vi "Resistivity of Bar sample Test.vi"(8 "error in (no error)":errorcluster) -> (0 "error out":errorcluster)   [LabVIEW 2016, in "Hall Effect Library.lvlib"]
doc: "This VI executes the Van Der Pauw Resisitivty Test and returns the voltage measurements V1-V8 taken during the test."
uses:
  Hall Effect Library.lvlib
  Controls/Measurement.ctl
  Public/Controls/Data Items.ctl
  Public/Controls/Tests.ctl
  Global Variables/Test Settings.vi
  Global Variables/Instrument Locations.vi
  Global Variables/Hall Effect Data.vi
panel:
  out "Soak Until":timestamp
  out "Measurement":T1
  out "Test Step":T2(ring)
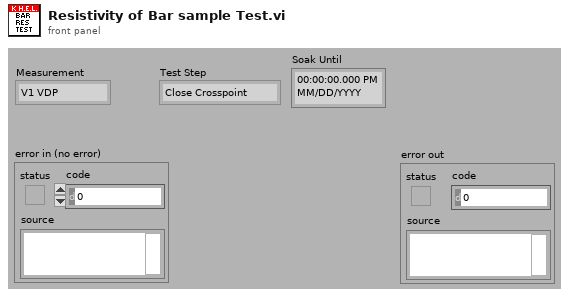
[diagram p1: front panel]
types:
  T1 = typedef "Hall Effect Library.lvlib/Measurement.ctl" = enum16{"V1 VDP", "V2 VDP", "V3 VDP", "V4 VDP", "V5 VDP", "V6 VDP", "V7 VDP", "V8 VDP", "V1 HE", "V2 HE", "V3 HE", "V4 HE", "V5 HE", "V6 HE", "V7 HE", "V8 HE", "V1 Res Bar", "V1 Hall Bar", "V1 Res 6-Cot", "V2 Res 6-Cot", "V3 Res 6-Cot", "V4 Res 6-Cot", "V1 Hall 6-Cot", "V2 Hall 6-Cot", "V3 Hall 6-Cot", "V4 Hall 6-Cot", "V5 Hall 6-Cot", "V6 Hall 6-Cot", "V7 Hall 6-Cot", "V8 Hall 6-Cot", "V1 Res 8-Cot", "V2 Res 8-Cot", "V3 Res 8-Cot", "V4 Res 8-Cot", "V1 Hall 8-Cot", "V2 Hall 8-Cot", "V3 Hall 8-Cot", "V4 Hall 8-Cot"}
  T2 = enum16{"Close Crosspoint", "Soak 1", "Zero Ammeter", "Zero Voltmeter", "I-SRC On", "Init Ammeter", "Soak 2", "Measure I", "Measure V", "I-SRC Off", "Open Crosspoint", "Done"}
  T3 = typedef "Hall Effect Library.lvlib/Resisitivity.ctl" = enum16{"Low", "High"}
  T4 = typedef "Hall Effect Library.lvlib/Tests.ctl" = enum16{"Van Der Pauw", "Hall Effect", "Bar Sample Resistivity", "Bar Sample Hall ", "6-Contact Sample Resistivity", "6-Contact Sample Hall", "8-Contact Sample Resistivity", "8-Contact Sample Hall", ""}
  T5 = typedef "Hall Effect Library.lvlib/Data Items.ctl" = enum16{"V1 Van Der Pauw", "V2 Van Der Pauw", "V3 Van Der Pauw", "V4 Van Der Pauw", "V5 Van Der Pauw", "V6 Van Der Pauw", "V7 Van Der Pauw", "V8 Van Der Pauw", "V1 Hall Effect", "V2 Hall Effect", "V3 Hall Effect", "V4 Hall Effect", "V5 Hall Effect", "V6  Hall Effect", "V7 Hall Effect", "V8 Hall Effect", "V1 Res Bar", "V1 Hall Bar", "V1 Res 6-Cot", "V2 Res 6-Cot", "V3 Res 6-Cot", "V4 Res 6-Cot", "V1 Hall 6-Cot", "V2 Hall 6-Cot", "V3 Hall 6-Cot", "V4 Hall 6-Cot", "V5 Hall 6-Cot", "V6 Hall 6-Cot", "V7 Hall 6-Cot", "V8 Hall 6-Cot", "V1 Res 8-Cot", "V2 Res 8-Cot", "V3 Res 8-Cot", "V4 Res 8-Cot", "V1 Hall 8-Cot", "V2 Hall 8-Cot", "V3 Hall 8-Cot", "V4 Hall 8-Cot", "Van Der Pauw Results", "Hall Effect Results", "Bar Sample Resistivity Results", "Bar Sample Hall Results", "6-Contact Resistivity Results", "6-Contact Hall Results", "8-Contact Resistivity Results", "8-Contact Hall Results"}
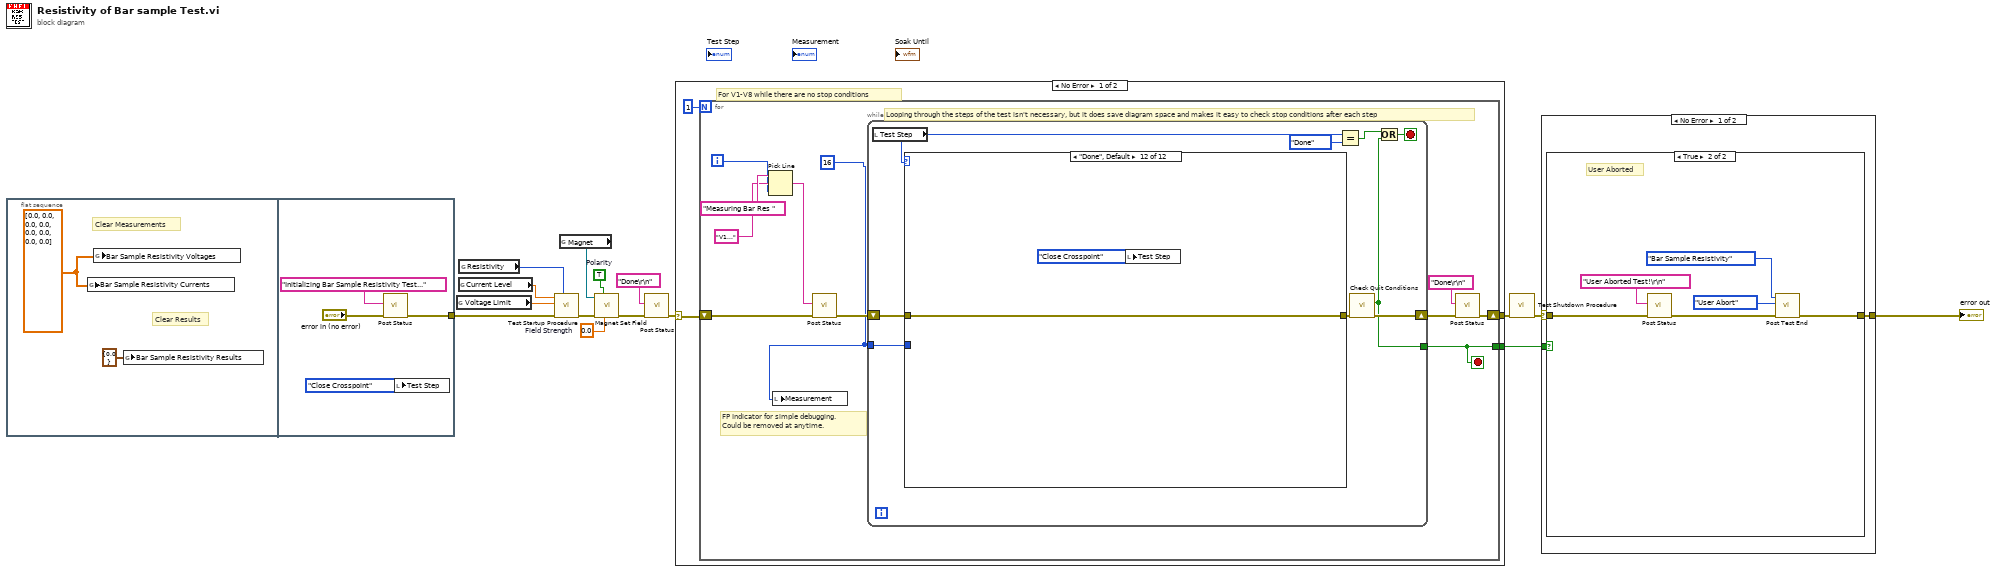
[diagram p0: block diagram]
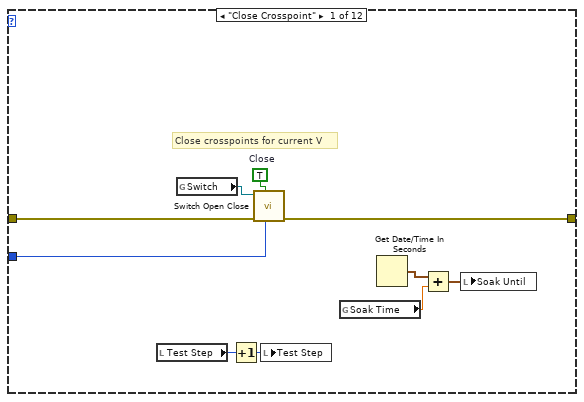
[diagram p2: hidden frame]
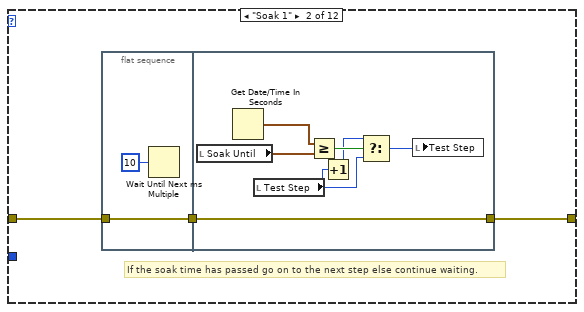
[diagram p3: hidden frame]
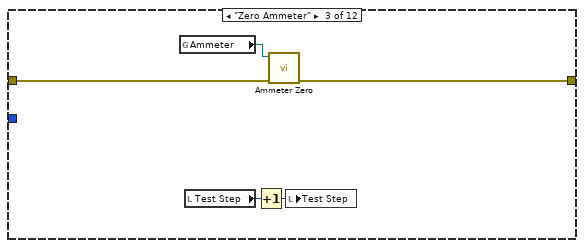
[diagram p4: hidden frame]
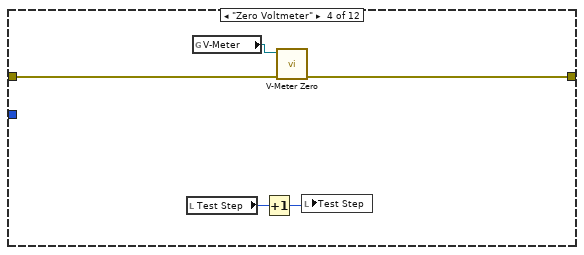
[diagram p5: hidden frame]
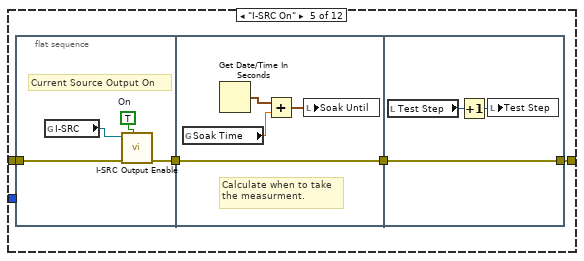
[diagram p6: hidden frame]
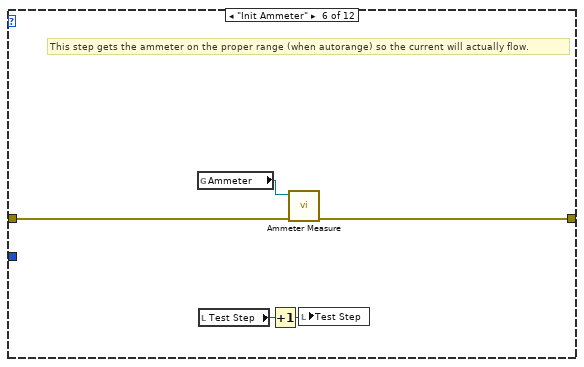
[diagram p7: hidden frame]
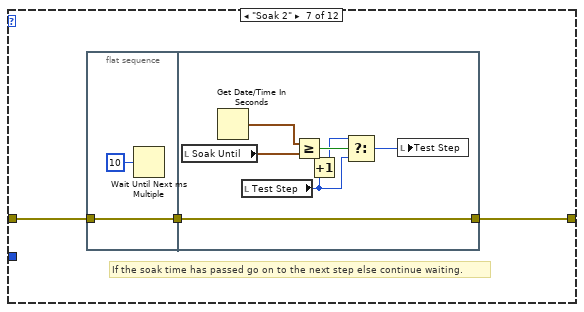
[diagram p8: hidden frame]
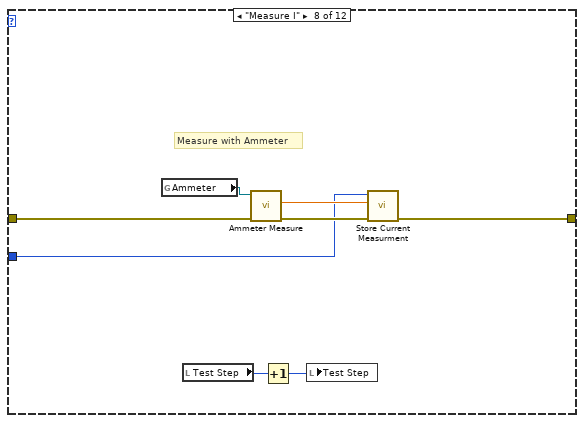
[diagram p9: hidden frame]
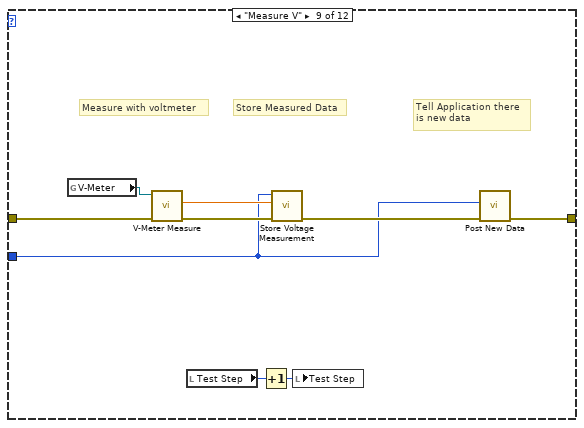
[diagram p10: hidden frame]
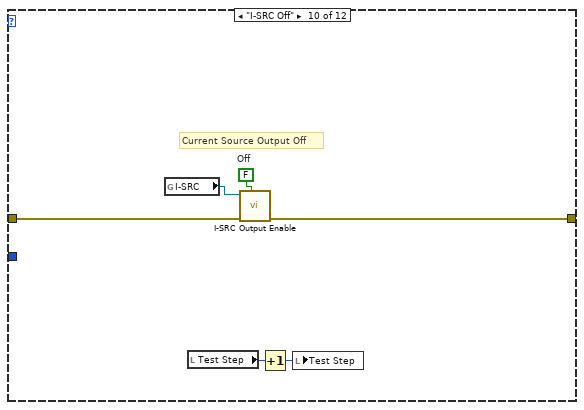
[diagram p11: hidden frame]
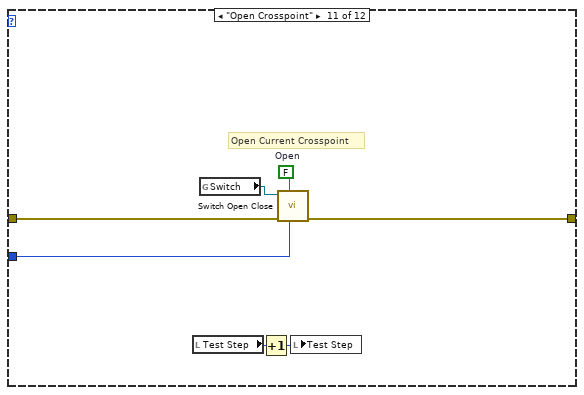
[diagram p12: hidden frame]
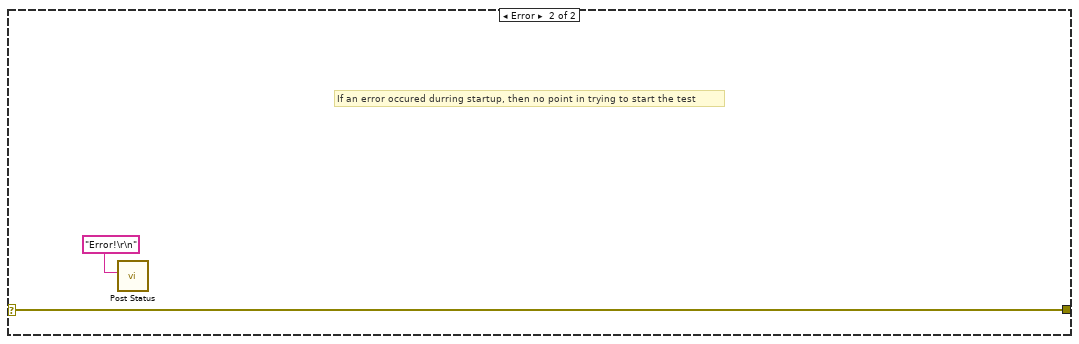
[diagram p13: hidden frame]
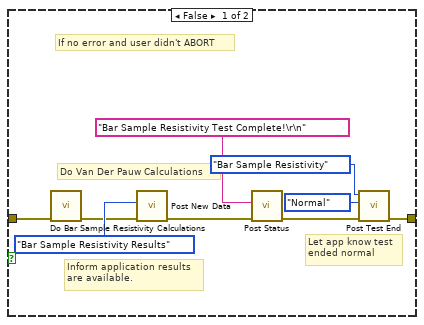
[diagram p14: hidden frame]
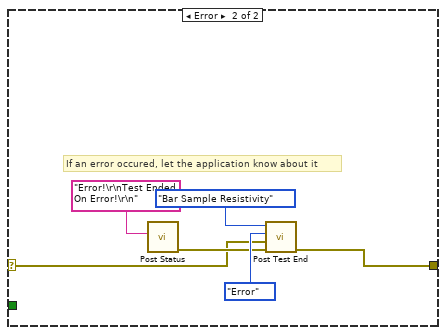
[diagram p15: hidden frame]
diagram:
  w4 = TRUE  # Polarity
  w5 = 0.0  # Field Strength
  n1 = flat-sequence {
    tunnel: [w21] -> w7
    frame #0 {
      w17 = dbl[] [0.0, 0.0, 0.0, 0.0, 0.0, 0.0, 0.0, 0.0] ("Van Der Pauw Voltages")
      # "Clear Results"
      # "Clear Measurements"
      n2 = global write "Hall Effect Data.vi" "Bar Sample Resistivity Currents"(w17) -> ()
      n3 = global write "Hall Effect Data.vi" "Bar Sample Resistivity Voltages"(w17) -> ()
      n4 = global write "Hall Effect Data.vi" "Bar Sample Resistivity Results"(cluster{"p":dbl} {"p"=0.0} ("Bar Sample Resistivity Results")) -> ()
    }
    frame #1 {
      n5 = call "Post Status.vi"("error in (no error)"="error in (no error)", "Status Message"="Initializing Bar Sample Resistivity Test...") -> ("error out"=w21:errorcluster)  [unwired: 9 out]
      n6 = local write "Test Step"(T2."Close Crosspoint" ("Test Step")) -> ()
    }
  }
  n7 = global read "Test Settings.vi" "Voltage Limit"() -> (w8:dbl)
  n8 = global read "Test Settings.vi" "Current Level"() -> (w9:dbl)
  n9 = global read "Test Settings.vi" "Resistivity"() -> (w10:T3)
  n10 = call "Test Startup Procedure.vi"("Resistivity"=w10, "error in (no error)"=w7, "Voltage Limit"=w8, "Current Level"=w9) -> ("error out"=w2:errorcluster)  [unwired: 7 out]
  n11 = global read "Instrument Locations.vi" "Magnet"() -> (w3:refnum<visa-resource-name>)
  n12 = call "Magnet Set Field.vi"("Field Strength"=w5, "Polarity"=w4, "error in (no error)"=w2, "VISA resource name in"=w3) -> ("error out"=w1:errorcluster)  [unwired: 7 out]
  n13 = call "Post Status.vi"("error in (no error)"=w1, "Status Message"="Done\r\n") -> ("error out"=w12:errorcluster)  [unwired: 9 out]
  n14 = case shown="No Error" w12 {
    selector: w12 -> [w23 w143]
    tunnel: [w25 w143] -> w11
    tunnel: [w24 _] -> w13
    frame No Error {
      # "For V1-V8 while there are no stop conditions"
      n15 = for {
        N: 1 -> [_]
        shift-right: [w29] -> w25
        shift-left: w23 -> [w32]
        tunnel: [w28] -> w24
        i -> [w27]
        stop <- w28 stop-if-true
        w26 = 16
        # "FP Indicator for simple debugging.\nCould be removed at anytime."
        # "Looping through the steps of the test isn't necessary, but it does save diagram space and makes it easy to check stop conditions after each step"
        n16 = Pick Line(string ("")="Measuring Bar Res ", multi-line string="V1...", line index=w27) -> (output string=w34:string)
        n17 = local write "Measurement"(w26) -> ()
        n18 = call "Post Status.vi"("error in (no error)"=w32, "Status Message"=w34) -> ("error out"=w33:errorcluster)  [unwired: 9 out]
        n19 = while {
          shift-right: [w43] -> w30
          shift-left: w33 -> [w45]
          tunnel: w26 -> [w44]
          tunnel: [w39] -> w28
          stop <- w42 stop-if-true
          n20 = local read "Test Step"() -> (w40:T2)
          n21 = case shown="\"Done\", Default" w40 {
            tunnel: [w53 w56 w70 w75 w80 w96 w99 w114 w121 w129 w137 w141] -> w38
            tunnel: w45 -> [w52 w57 w71 w76 w81 w97 w100 w116 w125 w130 w136 w141]
            tunnel: w44 -> [w51 _ _ _ _ _ _ w112 w120 _ w135 _]
            frame "Close Crosspoint" {
              w54 = TRUE  # Close
              # "Close crosspoints for current V"
              n22 = local read "Test Step"() -> (w47:T2)
              n23 = global read "Instrument Locations.vi" "Switch"() -> (w55:refnum<visa-resource-name>)
              n24 = Increment(x=w47) -> (x+1=w46:T2)
              n25 = call "Switch Open Close.vi"("Measurement"=w51, "Open/Close (F: Open)"=w54, "error in (no error)"=w52, "VISA resource name in"=w55) -> ("error out"=w53:errorcluster)  [unwired: 7 out]
              n26 = local write "Test Step"(w46) -> ()
              n27 = global read "Test Settings.vi" "Soak Time"() -> (w49:dbl)
              n28 = Get Date/Time In Seconds() -> (seconds since 1Jan1904=w48:timestamp)
              n29 = Add(x=w48, y=w49) -> (x+y=w50:timestamp)
              n30 = local write "Soak Until"(w50) -> ()
            }
            frame "Soak 1" {
              # "If the soak time has passed go on to the next step else continue waiting."
              n31 = flat-sequence {
                tunnel: w57 -> [w59]
                tunnel: [w59] -> w58
                tunnel: [w63] -> w56
                tunnel: w58 -> [w63]
                frame #0 {
                  n32 = Wait Until Next ms Multiple(millisecond multiple=u32 10) -> ()  [unwired: 1 out]
                }
                frame #1 {
                  n33 = local read "Soak Until"() -> (w66:timestamp)
                  n34 = Get Date/Time In Seconds() -> (seconds since 1Jan1904=w67:timestamp)
                  n35 = local read "Test Step"() -> (w62:T2)
                  n36 = Greater Or Equal?(x=w67, y=w66) -> (x >= y?=w65:bool)
                  n37 = Increment(x=w62) -> (x+1=w61:T2)
                  n38 = Select(t=w61, s=w65, f=w62) -> (s? t:f=w64:T2)
                  n39 = local write "Test Step"(w64) -> ()
                }
              }
            }
            frame "Zero Ammeter" {
              n40 = global read "Instrument Locations.vi" "Ammeter"() -> (w72:refnum<visa-resource-name>)
              n41 = local read "Test Step"() -> (w69:T2)
              n42 = Increment(x=w69) -> (x+1=w68:T2)
              n43 = call "Ammeter Zero.vi"("error in (no error)"=w71, "VISA resource name in"=w72) -> ("error out"=w70:errorcluster)  [unwired: 9 out]
              n44 = local write "Test Step"(w68) -> ()
            }
            frame "Zero Voltmeter" {
              n45 = local read "Test Step"() -> (w73:T2)
              n46 = global read "Instrument Locations.vi" "V-Meter"() -> (w77:refnum<visa-resource-name>)
              n47 = Increment(x=w73) -> (x+1=w74:T2)
              n48 = call "V-Meter Zero.vi"("error in (no error)"=w76, "VISA resource name in"=w77) -> ("error out"=w75:errorcluster)  [unwired: 9 out]
              n49 = local write "Test Step"(w74) -> ()
            }
            frame "I-SRC On" {
              n50 = flat-sequence {
                tunnel: w81 -> [w83]
                tunnel: [w82] -> w79
                tunnel: w79 -> [w89]
                tunnel: [w89] -> w78
                tunnel: [w92] -> w80
                tunnel: w78 -> [w92]
                frame #0 {
                  w84 = TRUE  # On
                  # "Current Source Output On"
                  n51 = global read "Instrument Locations.vi" "I-SRC"() -> (w85:refnum<visa-resource-name>)
                  n52 = call "I-SRC Output Enable.vi"("Output (Off)"=w84, "error in (no error)"=w83, "VISA resource name in"=w85) -> ("error out"=w82:errorcluster)  [unwired: 8 out]
                }
                frame #1 {
                  # "Calculate when to take\nthe measurment."
                  n53 = global read "Test Settings.vi" "Soak Time"() -> (w87:dbl)
                  n54 = Get Date/Time In Seconds() -> (seconds since 1Jan1904=w86:timestamp)
                  n55 = Add(x=w86, y=w87) -> (x+y=w88:timestamp)
                  n56 = local write "Soak Until"(w88) -> ()
                }
                frame #2 {
                  n57 = local read "Test Step"() -> (w91:T2)
                  n58 = Increment(x=w91) -> (x+1=w90:T2)
                  n59 = local write "Test Step"(w90) -> ()
                }
              }
            }
            frame "Init Ammeter" {
              # "This step gets the ammeter on the proper range (when autorange) so the current will actually flow."
              n60 = global read "Instrument Locations.vi" "Ammeter"() -> (w95:refnum<visa-resource-name>)
              n61 = local read "Test Step"() -> (w94:T2)
              n62 = Increment(x=w94) -> (x+1=w93:T2)
              n63 = call "Ammeter Measure.vi"("error in (no error)"=w97, "VISA resource name in"=w95) -> ("error out"=w96:errorcluster)  [unwired: 9 out]
              n64 = local write "Test Step"(w93) -> ()
            }
            frame "Soak 2" {
              # "If the soak time has passed go on to the next step else continue waiting."
              n65 = flat-sequence {
                tunnel: w100 -> [w101]
                tunnel: [w101] -> w98
                tunnel: [w105] -> w99
                tunnel: w98 -> [w105]
                frame #0 {
                  n66 = Wait Until Next ms Multiple(millisecond multiple=u32 10) -> ()  [unwired: 1 out]
                }
                frame #1 {
                  n67 = local read "Soak Until"() -> (w108:timestamp)
                  n68 = Get Date/Time In Seconds() -> (seconds since 1Jan1904=w109:timestamp)
                  n69 = local read "Test Step"() -> (w103:T2)
                  n70 = Greater Or Equal?(x=w109, y=w108) -> (x >= y?=w107:bool)
                  n71 = Increment(x=w103) -> (x+1=w104:T2)
                  n72 = Select(t=w104, s=w107, f=w103) -> (s? t:f=w106:T2)
                  n73 = local write "Test Step"(w106) -> ()
                }
              }
            }
            frame "Measure I" {
              # "Measure with Ammeter"
              n74 = global read "Instrument Locations.vi" "Ammeter"() -> (w117:refnum<visa-resource-name>)
              n75 = local read "Test Step"() -> (w111:T2)
              n76 = call "Ammeter Measure.vi"("error in (no error)"=w116, "VISA resource name in"=w117) -> ("error out"=w115:errorcluster, "Measurement"=w113:dbl)  [unwired: 8 out]
              n77 = Increment(x=w111) -> (x+1=w110:T2)
              n78 = local write "Test Step"(w110) -> ()
              n79 = call "Store Current Measurment.vi"("error in"=w115, "Value"=w113, "Measurement"=w112) -> ("error out"=w114:errorcluster)  [unwired: 8 out]
            }
            frame "Measure V" {
              # "Tell Application there\nis new data"
              # "Store Measured Data"
              # "Measure with voltmeter"
              n80 = global read "Instrument Locations.vi" "V-Meter"() -> (w126:refnum<visa-resource-name>)
              n81 = call "V-Meter Measure.vi"("error in (no error)"=w125, "VISA resource name in"=w126) -> ("error out"=w124:errorcluster, "Measurement"=w123:dbl)  [unwired: 1 in, 7 out]
              n82 = local read "Test Step"() -> (w119:T2)
              n83 = Increment(x=w119) -> (x+1=w118:T2)
              n84 = call "Store Voltage Measurement.vi"("error in"=w124, "Value"=w123, "Measurement"=w120) -> ("error out"=w122:errorcluster)  [unwired: 8 out]
              n85 = local write "Test Step"(w118) -> ()
              n86 = call "Post New Data.vi"("error in (no error)"=w122, "Data Item"=w120) -> ("error out"=w121:errorcluster)  [unwired: 9 out]
            }
            frame "I-SRC Off" {
              w131 = FALSE  # Off
              # "Current Source Output Off"
              n87 = global read "Instrument Locations.vi" "I-SRC"() -> (w132:refnum<visa-resource-name>)
              n88 = local read "Test Step"() -> (w128:T2)
              n89 = call "I-SRC Output Enable.vi"("Output (Off)"=w131, "error in (no error)"=w130, "VISA resource name in"=w132) -> ("error out"=w129:errorcluster)  [unwired: 8 out]
              n90 = Increment(x=w128) -> (x+1=w127:T2)
              n91 = local write "Test Step"(w127) -> ()
            }
            frame "Open Crosspoint" {
              w138 = FALSE  # Open
              # "Open Current Crosspoint"
              n92 = local read "Test Step"() -> (w133:T2)
              n93 = global read "Instrument Locations.vi" "Switch"() -> (w139:refnum<visa-resource-name>)
              n94 = Increment(x=w133) -> (x+1=w134:T2)
              n95 = call "Switch Open Close.vi"("Measurement"=w135, "Open/Close (F: Open)"=w138, "error in (no error)"=w136, "VISA resource name in"=w139) -> ("error out"=w137:errorcluster)  [unwired: 7 out]
              n96 = local write "Test Step"(w134) -> ()
            }
            frame "Done", Default {
              n97 = local write "Test Step"(T2."Close Crosspoint" ("Test Step")) -> ()
            }
          }
          n98 = Equal?(x=w40, y=T2."Done") -> (x = y?=w41:bool)
          n99 = call "Check Quit Conditions.vi"("error in (no error)"=w38) -> ("error out"=w43:errorcluster, "Quit?"=w39:bool)  [unwired: 9 out]
          n100 = Or(x=w41, y=w39) -> (x .or. y?=w42:bool)
        }
        n101 = call "Post Status.vi"("error in (no error)"=w30, "Status Message"="Done\r\n") -> ("error out"=w29:errorcluster)  [unwired: 9 out]
      }
    }
    frame Error {
      # "If an error occured durring startup, then no point in trying to start the test"
      n102 = call "Post Status.vi"("Status Message"="Error!\r\n") -> ()  [unwired: 1 in, 10 out]
    }
  }
  n103 = call "Test Shutdown Procedure.vi"("error in (no error)"=w11) -> ("error out"=w14:errorcluster)  [unwired: 10 out]
  n104 = case shown="No Error" w14 {
    selector: w14 -> [w145 w163]
    tunnel: w13 -> [w146 _]
    tunnel: [w144 w165] -> w15
    frame No Error {
      n105 = case shown="True" w146 {
        tunnel: w145 -> [w148 w160]
        tunnel: [w151 w157] -> w144
        frame False {
          # "Let app know test\nended normal"
          # "Inform application results\nare available."
          # "Do Van Der Pauw Calculations"
          # "If no error and user didn't ABORT"
          n106 = call "Do Bar Sample Resistivity Calculations.vi"("error in (no error)"=w148) -> ("error out"=w147:errorcluster)  [unwired: 10 in]
          n107 = call "Post New Data.vi"("error in (no error)"=w147, "Data Item"=Data_Items."Bar Sample Resistivity Results") -> ("error out"=w153:errorcluster)  [unwired: 9 out]
          n108 = call "Post Status.vi"("error in (no error)"=w153, "Status Message"="Bar Sample Resistivity Test Complete!\r\n") -> ("error out"=w150:errorcluster)  [unwired: 9 out]
          n109 = call "Post Test End.vi"("error in (no error)"=w150, "Test End"=enum16{"Normal", "User Abort", "Error"}."Normal", "Test"=Tests."Bar Sample Resistivity") -> ("error out"=w151:errorcluster)  [unwired: 1 in, 7 out]
        }
        frame True {
          # "User Aborted"
          n110 = call "Post Status.vi"("error in (no error)"=w160, "Status Message"="User Aborted Test!\r\n") -> ("error out"=w159:errorcluster)  [unwired: 9 out]
          n111 = call "Post Test End.vi"("error in (no error)"=w159, "Test End"=enum16{"Normal", "User Abort", "Error"}."User Abort", "Test"=Tests."Bar Sample Resistivity") -> ("error out"=w157:errorcluster)  [unwired: 1 in, 7 out]
        }
      }
    }
    frame Error {
      # "If an error occured, let the application know about it"
      n112 = call "Post Status.vi"("Status Message"="Error!\r\nTest Ended On Error!\r\n") -> ("error out"=w164:errorcluster)  [unwired: 1 in, 9 out]
      n113 = call "Post Test End.vi"("error in (no error)"=w164, "Test End Error (no error)"=w163, "Test End"=enum16{"Normal", "User Abort", "Error"}."Error", "Test"=Tests."Bar Sample Resistivity") -> ("error out"=w165:errorcluster)  [unwired: 7 out]
    }
  }
  "error out" <- w15
